vi "GenerateDefaultSubpanels.vi"(8 "error in (no error)":errorcluster, 10 "Number":i32, 11 "SMO.UI.MAUI in":refnum<class "SMO.UI.MAUI.lvclass">) -> (0 "error out":errorcluster, 2 "Array":refnum<class "SMO.UI.Embedded.lvclass">[](array[class]), 3 "SMO.UI.MAUI out":refnum<class "SMO.UI.MAUI.lvclass">)   [LabVIEW 2020, in "SMO.UI.MAUI.lvclass"]
uses:
  SMO.UI.MAUI.lvclass
  <vilib>/Levylab/SMO.UI.Embedded/SMO.UI.Embedded.lvclass
  <vilib>/JKI/JKI SMO/SMO/SMO.lvclass
  C:/Program Files (x86)/National Instruments/LabVIEW 2020/vi.lib/JKI/JKI SMO/SMO.UI/SMO.UI.lvclass
  C:/Program Files (x86)/National Instruments/LabVIEW 2020/vi.lib/JKI/JKI SMO/SMO/SMO.lvclass
  C:/Program Files (x86)/National Instruments/LabVIEW 2020/vi.lib/Levylab/SMO.UI.Embedded/SMO.UI.Embedded.lvclass
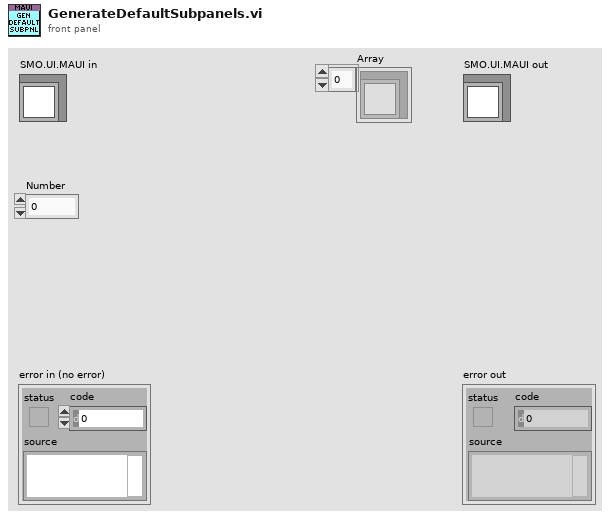
[diagram p1: front panel]
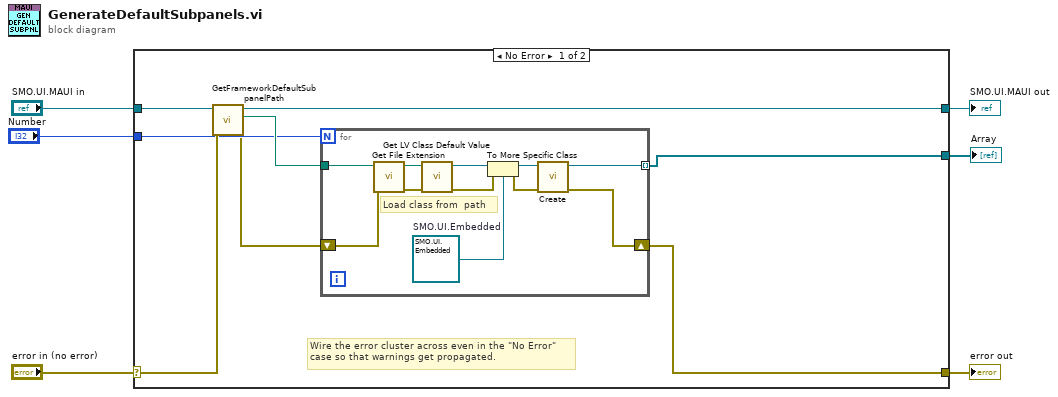
[diagram p0: block diagram]
diagram:
  n1 = case shown="No Error" "error in (no error)" {
    selector: "error in (no error)" -> [w13 w27]
    tunnel: [w9 w27] -> w5
    tunnel: [w8 w26] -> w3
    tunnel: "SMO.UI.MAUI in" -> [w14 w26]
    tunnel: "Number" -> [w11 _]
    tunnel: [w7 _] -> w1
    frame No Error {
      # "Wire the error cluster across even in the \"No Error\"\ncase so that warnings get propagated."
      n2 = call "GetFrameworkDefaultSubpanelPath.vi"("error in (no error)"=w13, "SMO.UI.MAUI in"=w14) -> ("error out"=w10:errorcluster, "path"=w12:path, "SMO.UI.MAUI out"=w8:refnum<class "SMO.UI.MAUI.lvclass">)  [unwired: 7 in]
      n3 = for {
        N: w11 -> [_]
        tunnel: w12 -> [w20]
        tunnel: [w16] -> w7 mode=indexing
        shift-right: [w15] -> w9
        shift-left: w10 -> [w19]
        w21 = refnum<class "SMO.UI.Embedded.lvclass"> refnum  # SMO.UI.Embedded
        # "Load class from  path"
        n4 = call <vilib>:"Get File Extension.vi"("error in (no error)"=w19, "file"=w20) -> ("error out"=w24:errorcluster, "dup file"=w22:path)  [unwired: 5 in, 3 out]
        n5 = call <vilib>:"Get LV Class Default Value.vi"("error in (no error)"=w24, "class path"=w22) -> ("error out"=w25:errorcluster, "object"=w23:refnum<class>)  [unwired: 8 in]
        n6 = To More Specific Class(target class=w21, reference=w23, error in=w25) -> (specific class reference=w18:refnum<class "SMO.UI.Embedded.lvclass">, error out=w17:errorcluster)
        n7 = call <vilib>:"Create.vi"("error in (no error)"=w17, "SMO"=w18) -> ("error out"=w15:errorcluster, "SMO out"=w16:refnum<class "SMO.UI.Embedded.lvclass">)  [unwired: 7 in, 1 out]
      }
    }
    frame Error {
    }
  }
  "error out" <- w5
  "SMO.UI.MAUI out" <- w3
  "Array" <- w1
